vi "MCLB_FocusName_Tests.vi"(11 "error in":errorcluster) -> (15 "error out":errorcluster)   [LabVIEW 2016, in "DronaTest.lvlib"]
uses:
  DronaTest.lvlib
  APIs/Stimulus/ControlValue/SetValueAuto.vi
  APIs/Stimulus/ControlValue/Controls/MC Listbox/SetValueByItemName.vi
  APIs/Assert/AssertControlValue/Controls/MC Listbox/AssertValueByFocusName.vi
  <vilib>/addons/_JKI Toolkits/Caraya/classes/Assert/Assert Error.vi
  <vilib>/addons/_JKI Toolkits/Caraya/classes/Assert/Assert Equal Value_Variant.vi
  <vilib>/addons/_JKI Toolkits/Caraya/classes/Test/Test.lvclass
  Drona.lvlib
  <vilib>/SLL Toolkit/SLL Debug/SLL Debug.lvlib
  APIs/Stimulus/ControlValue/ControlValue.lvlib
  <vilib>/addons/_JKI Toolkits/Caraya/classes/Assert/Assert.lvclass
  APIs/Stimulus/ControlValue/Controls/MC Listbox/StimulusMCListbox.lvlib
  APIs/Assert/AssertControlValue/Controls/MC Listbox/AssertMCListbox.lvlib
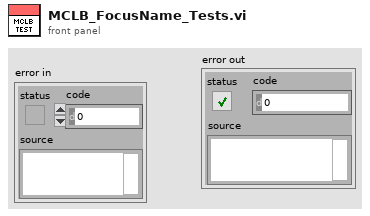
[diagram p1: front panel]
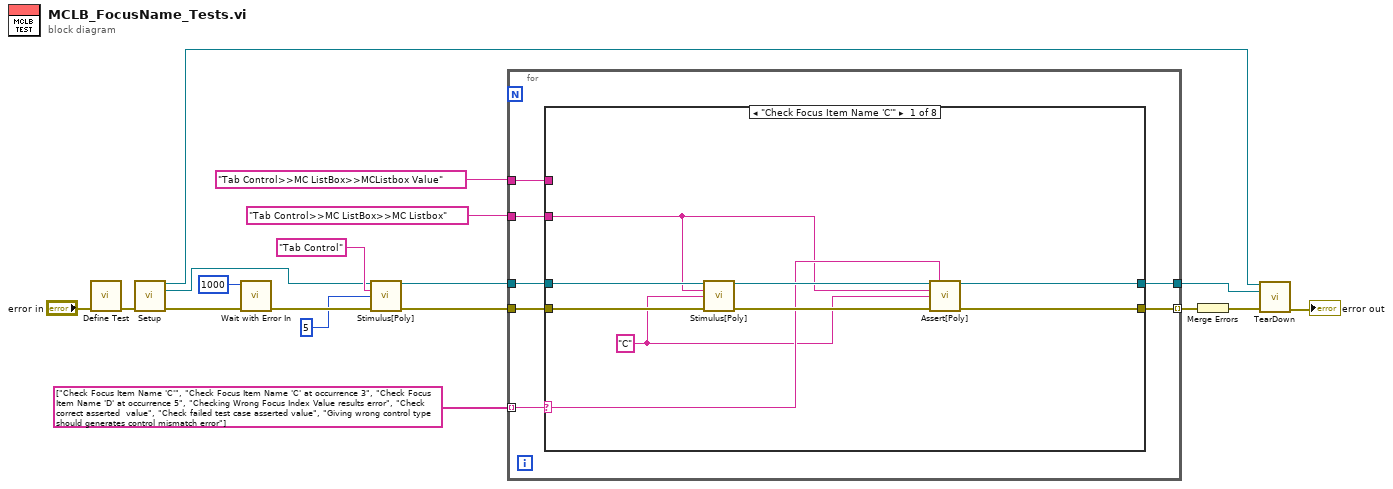
[diagram p0: block diagram]
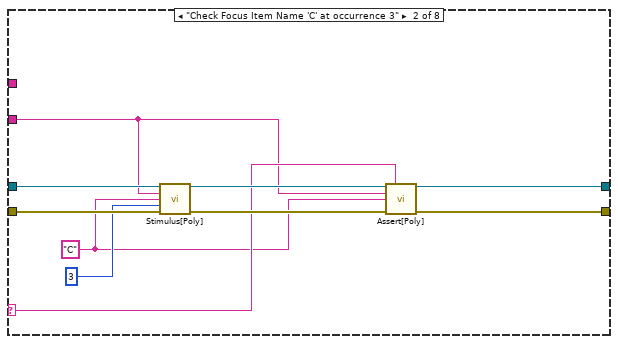
[diagram p2: hidden frame]
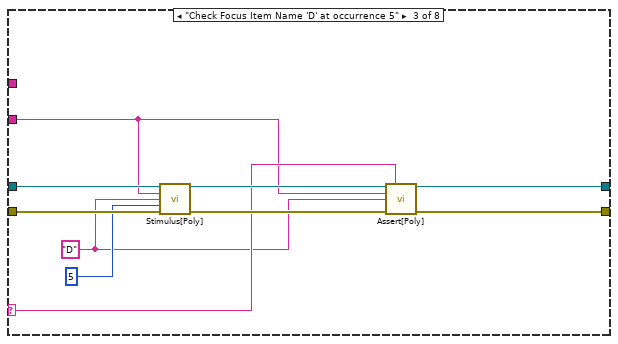
[diagram p3: hidden frame]
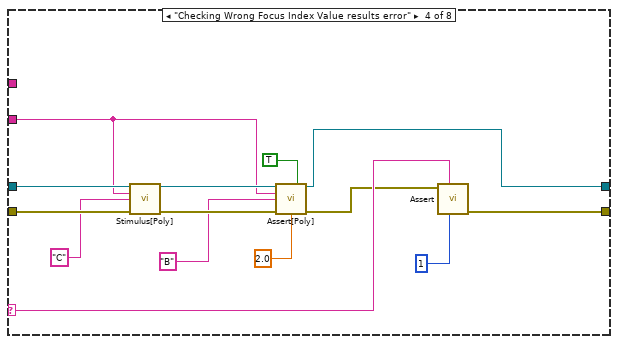
[diagram p4: hidden frame]
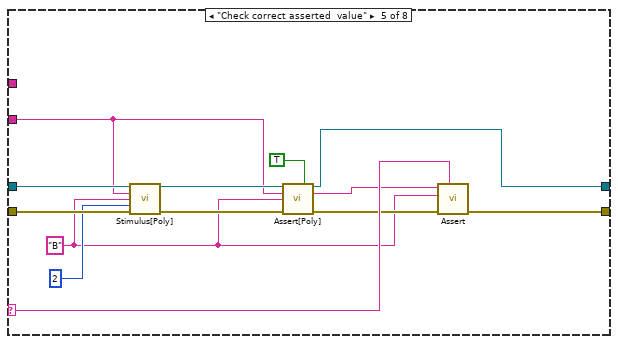
[diagram p5: hidden frame]
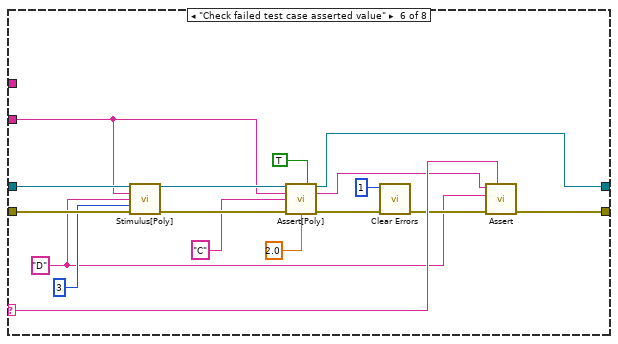
[diagram p6: hidden frame]
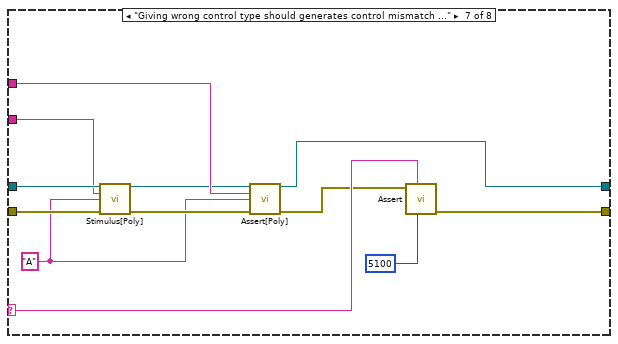
[diagram p7: hidden frame]
diagram:
  n1 = call <vilib>:"Define Test.vi"("error in (no error)"="error in") -> ("error out"=w9:errorcluster)  [unwired: 9 in, 1 out]
  n2 = call "Setup.vi"("error in (no error)"=w9) -> ("Application Ref"=w5:refnum<vi>, "VI out"=w7:refnum<vi>, "error out"=w8:errorcluster)  [unwired: 12 in]
  n3 = call <vilib>:"Wait with Error In.vi"("error in (no error)"=w8, "milliseconds to wait"=u32 1000) -> ("error out"=w16:errorcluster)  [unwired: 9 in]
  n4 = call-poly "Stimulus[Poly].vi"("VI Reference In"=w7, "Control Path"="Tab Control", "Value (Signaling)"=5, "error in"=w16) -> ("VI Reference Out"=w12:refnum<vi>, "error out"=w15:errorcluster)  [unwired: 10 in]
  n5 = for {
    tunnel: w12 -> [w24]
    tunnel: "Tab Control>>MC ListBox>>MC Listbox" ("Control Path") -> [w23]
    tunnel: "Tab Control>>MC ListBox>>MCListbox Value" ("Control Path") -> [w22]
    tunnel: string[] ["Check Focus Item Name 'C'", "Check Focus Item Name 'C' at occurrence 3", "Check Focus Item Name 'D' at occurrence 5", "Checking Wrong Focus Index Value results error", "Check correct asserted  value", "Check failed test case asserted value", "Giving wrong control type should generates control mismatch error"] -> [w20] mode=indexing
    tunnel: [w19] -> w4
    tunnel: w15 -> [w25]
    tunnel: [w21] -> w10 mode=indexing
    n6 = case shown="\"Check Focus Item Name 'C'\"" w20 {
      selector: w20 -> [w28 w38 w48 w67 w80 w97 w109 _]
      tunnel: w25 -> [w34 w44 w54 w65 w79 w96 w104 w112]
      tunnel: w24 -> [w33 w43 w53 w64 w78 w95 w102 w111]
      tunnel: w23 -> [w27 w37 w47 w61 w75 w92 w100 _]
      tunnel: w22 -> [_ _ _ _ _ _ w106 _]
      tunnel: [w30 w40 w50 w68 w81 w98 w110 w112] -> w21
      tunnel: [w29 w39 w49 w60 w74 w91 w105 w111] -> w19
      frame "Check Focus Item Name 'C'" {
        w26 = "C"
        n7 = call-poly "Stimulus[Poly].vi"("VI Reference In"=w33, "Control Path"=w27, "Item Name"=w26, "Error In"=w34) -> ("VI Reference Out"=w31:refnum<vi>, "Error Out"=w32:errorcluster)  [unwired: 10 in]
        n8 = call-poly "Assert[Poly].vi"("VI Reference In"=w31, "Test Label"=w28, "Control Path"=w27, "Item Name"=w26, "Error In"=w32) -> ("VI Reference Out"=w29:refnum<vi>, "Error Out"=w30:errorcluster)  [unwired: 8 in, 1 out]
      }
      frame "Check Focus Item Name 'C' at occurrence 3" {
        w35 = "C" ("Item Name")
        n9 = call-poly "Stimulus[Poly].vi"("VI Reference In"=w43, "Control Path"=w37, "Item Name"=w35, "Occurrence"=3 ("Item Index"), "Error In"=w44) -> ("VI Reference Out"=w41:refnum<vi>, "Error Out"=w42:errorcluster)  [unwired: 9 in]
        n10 = call-poly "Assert[Poly].vi"("VI Reference In"=w41, "Test Label"=w38, "Control Path"=w37, "Item Name"=w35, "Error In"=w42) -> ("VI Reference Out"=w39:refnum<vi>, "Error Out"=w40:errorcluster)  [unwired: 8 in, 1 out]
      }
      frame "Check Focus Item Name 'D' at occurrence 5" {
        w45 = "D" ("Item Name")
        n11 = call-poly "Stimulus[Poly].vi"("VI Reference In"=w53, "Control Path"=w47, "Item Name"=w45, "Occurrence"=5 ("Item Index"), "Error In"=w54) -> ("VI Reference Out"=w51:refnum<vi>, "Error Out"=w52:errorcluster)  [unwired: 9 in]
        n12 = call-poly "Assert[Poly].vi"("VI Reference In"=w51, "Test Label"=w48, "Control Path"=w47, "Item Name"=w45, "Error In"=w52) -> ("VI Reference Out"=w49:refnum<vi>, "Error Out"=w50:errorcluster)  [unwired: 8 in, 1 out]
      }
      frame "Checking Wrong Focus Index Value results error" {
        n13 = call-poly "Stimulus[Poly].vi"("VI Reference In"=w64, "Control Path"=w61, "Item Name"="C", "Error In"=w65) -> ("VI Reference Out"=w62:refnum<vi>, "Error Out"=w63:errorcluster)  [unwired: 10 in]
        n14 = call-poly "Assert[Poly].vi"("VI Reference In"=w62, "Assert Only? (F)"=TRUE, "Control Path"=w61, "Item Name"="B", "Error In"=w63, "Timeout(5 sec)"=2.0) -> ("VI Reference Out"=w60:refnum<vi>, "Error Out"=w59:errorcluster)  [unwired: 7 in, 1 out]
        n15 = call-poly <vilib>:"Assert.vi"("error code (1)"=1, "Label"=w67, "Error?"=w59) -> ("error out"=w68:errorcluster)  [unwired: 7 in, 1 out]
      }
      frame "Check correct asserted  value" {
        w70 = "B" ("Item Name")
        n16 = call-poly "Stimulus[Poly].vi"("VI Reference In"=w78, "Control Path"=w75, "Item Name"=w70, "Occurrence"=2, "Error In"=w79) -> ("VI Reference Out"=w76:refnum<vi>, "Error Out"=w77:errorcluster)  [unwired: 9 in]
        n17 = call-poly "Assert[Poly].vi"("VI Reference In"=w76, "Assert Only? (F)"=TRUE, "Control Path"=w75, "Item Name"=w70, "Error In"=w77) -> ("VI Reference Out"=w74:refnum<vi>, "Asserted Value"=w72:string, "Error Out"=w73:errorcluster)  [unwired: 8 in]
        n18 = call-poly <vilib>:"Assert.vi"("Label"=w80, "error in (no error)"=w73, "Y"=w70, "X"=w72) -> ("error out"=w81:errorcluster)  [unwired: 6 in, 1 out]
      }
      frame "Check failed test case asserted value" {
        w82 = "D" ("Item Name")
        n19 = call-poly "Stimulus[Poly].vi"("VI Reference In"=w95, "Control Path"=w92, "Item Name"=w82, "Occurrence"=3, "Error In"=w96) -> ("VI Reference Out"=w93:refnum<vi>, "Error Out"=w94:errorcluster)  [unwired: 9 in]
        n20 = call-poly "Assert[Poly].vi"("VI Reference In"=w93, "Assert Only? (F)"=TRUE, "Control Path"=w92, "Item Name"="C", "Error In"=w94, "Timeout(5 sec)"=2.0) -> ("VI Reference Out"=w91:refnum<vi>, "Asserted Value"=w85:string, "Error Out"=w90:errorcluster)  [unwired: 7 in]
        n21 = call <vilib>:"Clear Errors.vi"("error in (no error)"=w90, "specific error code to clear (0: all)"=1) -> ("error out"=w87:errorcluster)  [unwired: 4 in, 1 out]
        n22 = call-poly <vilib>:"Assert.vi"("Label"=w97, "error in (no error)"=w87, "Y"=w82, "X"=w85) -> ("error out"=w98:errorcluster)  [unwired: 6 in, 1 out]
      }
      frame "Giving wrong control type should generates control mismatch error" {
        w99 = "A" ("Item Name")
        n23 = call-poly "Stimulus[Poly].vi"("VI Reference In"=w102, "Control Path"=w100, "Item Name"=w99, "Error In"=w104) -> ("VI Reference Out"=w101:refnum<vi>, "Error Out"=w103:errorcluster)  [unwired: 10 in]
        n24 = call-poly "Assert[Poly].vi"("VI Reference In"=w101, "Control Path"=w106, "Item Name"=w99, "Error In"=w103) -> ("VI Reference Out"=w105:refnum<vi>, "Error Out"=w107:errorcluster)  [unwired: 9 in, 1 out]
        n25 = call-poly <vilib>:"Assert.vi"("error code (1)"=5100, "Label"=w109, "Error?"=w107) -> ("error out"=w110:errorcluster)  [unwired: 7 in, 1 out]
      }
      frame Default {
      }
    }
  }
  n26 = Merge Errors(w10) -> (w6:errorcluster)
  n27 = call "TearDown.vi"("Application Ref"=w5, "VI in"=w4, "error in (no error)"=w6) -> ("error out"=→"error out":errorcluster)  [unwired: 12 in]
